vi "midiInClose.vi"(8 "error in":errorcluster, 11 "midi in":refnum<class "midi.lvclass">) -> (0 "error out":errorcluster, 3 "midi out":refnum<class "midi.lvclass">)   [LabVIEW 2020, in "midi.lvclass"]
doc: "The midiInClose function closes the specified MIDI input device."
uses:
  midi.lvclass
  midi.lvclass/midi.ctl
  winmm.dll
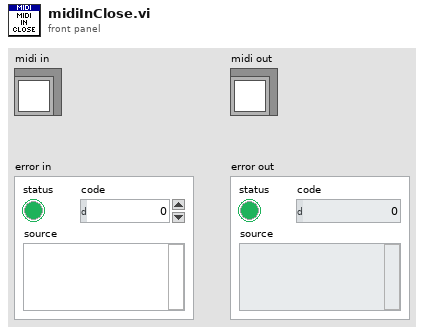
[diagram p1: front panel]
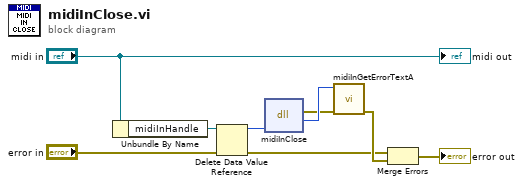
[diagram p0: block diagram]
diagram:
  n1 = Unbundle By Name("midi in") -> ("midiInHandle"=w4:refnum<data-value>)
  n2 = Delete Data Value Reference(data value reference=w4, error in="error in") -> (data value=w3:u64, error out=w1:errorcluster)
  n3 = dll-call lib="winmm.dll" fn="midiInClose"("hmi"=w3) -> (error out=w8:errorcluster, "return type"=w9:i32)  [unwired: 4 in, 1 out]
  n4 = call "midiInGetErrorTextA.vi"("error in"=w8, "Error Code"=w9) -> ("error out"=w6:errorcluster)  [unwired: 9 in]
  n5 = Merge Errors(w1, w6) -> (→"error out":errorcluster)
  "midi out" <- "midi in"
